vi "GetAiChans.vi"(6 "TimeOut":i32=1000, 8 "错误输入（无错误）":errorcluster, 9 "Num":u32, 10 "ChanSel":u16, 11 "DevIndex":i32) -> (0 "错误输出":errorcluster, 1 "FiFo Free":i32, 2 "Ai":sgl[][](array[numeric]), 3 "DevIndex Output":i32)   [LabVIEW 2018]
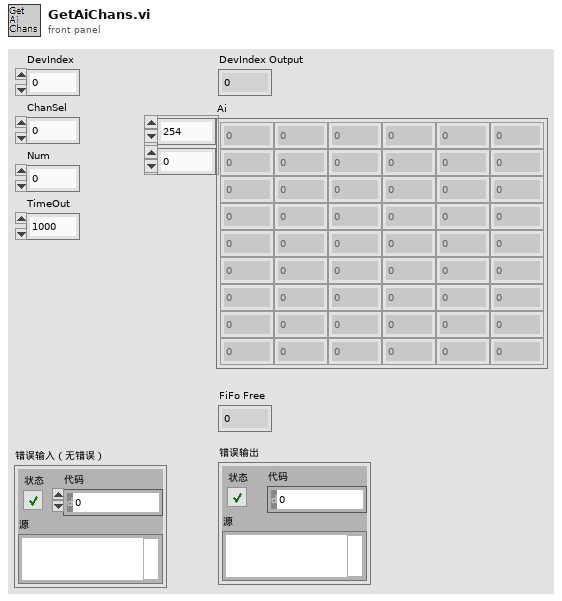
[diagram p1: front panel]
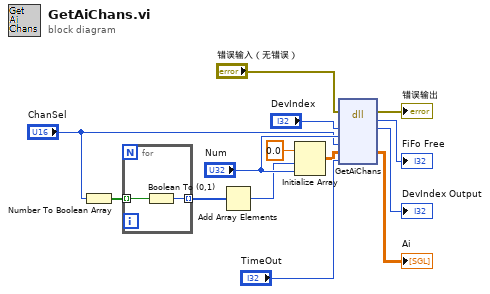
[diagram p0: block diagram]
diagram:
  n1 = Number To Boolean Array(number="ChanSel") -> (Boolean array=w3:bool[])
  n2 = for {
    tunnel: w3 -> [w16] mode=indexing
    tunnel: [w15] -> w2 mode=indexing
    n3 = Boolean To (0,1)(Boolean=w16) -> (0, 1=w15:i16)
  }
  n4 = Add Array Elements(numeric array=w2) -> (sum=w1:i16)
  n5 = Initialize Array(sgl 0.0 ("元素"), w1, "Num") -> (w9:sgl[][])
  n6 = dll-call lib="PTH2@abs H科研项目仅一项目程序32位usb-1000.dll" fn="GetAiChans"(error in="错误输入（无错误）", "DevIndex"="DevIndex", "Num"="Num", "ChanSel"="ChanSel", "Ai"=w9, "TimeOut"="TimeOut") -> (error out=→"错误输出":errorcluster, "FifoFree"=→"FiFo Free":i32, "DevIndex"=→"DevIndex Output":i32, "Ai"=→"Ai":sgl[][])  [unwired: 5 in, 1 out]
